vi "Execute.vi"(8 "error in":errorcluster, 9 "Consumer Queues in":T2, 10 "Trig Process Command in":refnum<class "TRIG Next Acq Request.lvclass">, 11 "Trig Process Data in":T1) -> (0 "error out":errorcluster, 1 "Consumer Queues out":T2, 2 "Stop?":bool, 3 "Trig Process Data out":T1)   [LabVIEW 2019, in "Trig Process.lvlib" / "TRIG Next Acq Request.lvclass"]
uses:
  TRIG Next Acq Request.lvclass
  TS Framework/Consumer Queues.ctl
  UI Process/Generic UI Command/Generic UI Process Command.lvclass
  DAC Process/Generic DAC Command/Generic DAC Process Command.lvclass
  Generic Trig Command/Generic Trig Process Command.lvclass
  Trig Process Data.ctl
  DAC Process/Start DAC/Start DAC.lvclass
  DAC Process/Start DAC/Start DAC.lvclass/Start DAC.ctl
  TS Framework/TS Framework.lvlib
  Trig Process.lvlib
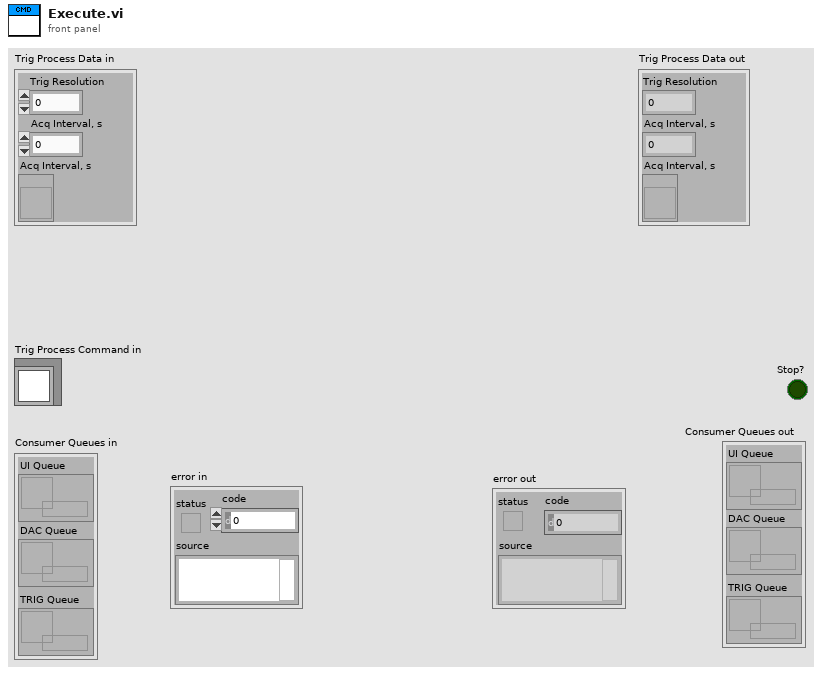
[diagram p1: front panel]
types:
  T1 = typedef "Trig Process.lvlib/Trig Process Data.ctl" = cluster{"Trig Resolution":u32, "Ctrl Interval":dbl, "Acq Interval":refnum<vi>}
  T2 = typedef "TS Framework.lvlib/Consumer Queues.ctl" = cluster{"UI Queue":refnum<queue>, "DAC Queue":refnum<queue>, "TRIG Queue":refnum<queue>}
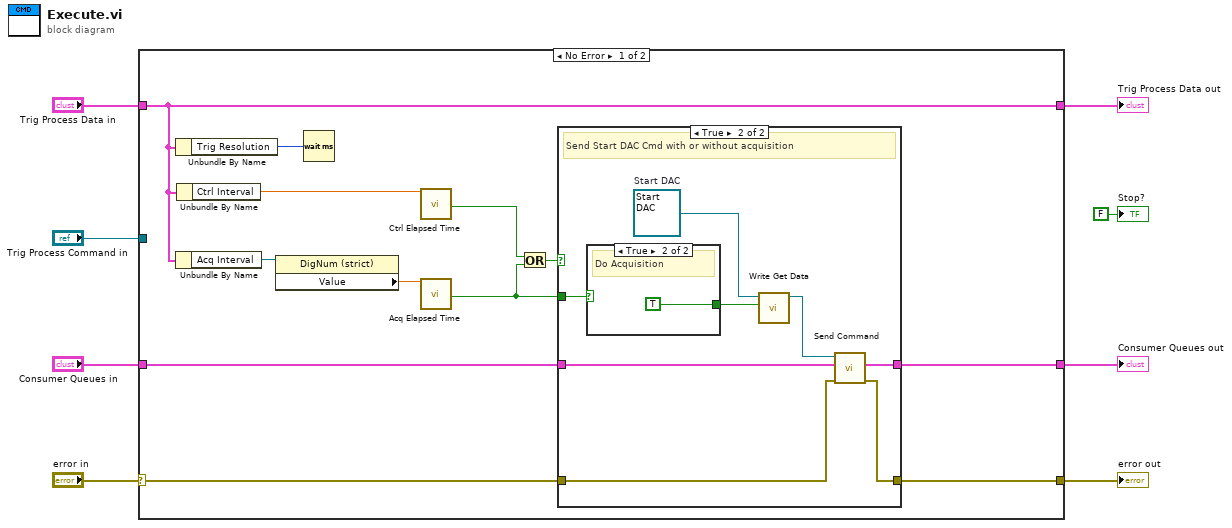
[diagram p0: block diagram]
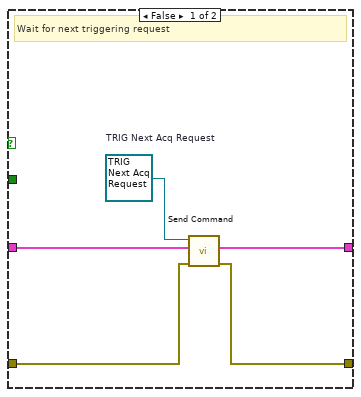
[diagram p2: hidden frame]
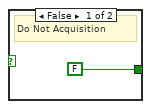
[diagram p3: hidden frame]
diagram:
  n1 = case shown="No Error" "error in" {
    selector: "error in" -> [w10 w38]
    tunnel: [w9 w38] -> w3
    tunnel: "Consumer Queues in" -> [w20 w37]
    tunnel: [w19 w37] -> w4
    tunnel: "Trig Process Data in" -> [w15 w36]
    tunnel: [w15 w36] -> w5
    tunnel: "Trig Process Command in" -> [_ _]
    frame No Error {
      n2 = Unbundle By Name(w15) -> ("Trig Resolution"=w17:u32)
      n3 = Unbundle By Name(w15) -> ("Acq Interval"=w14:refnum<vi>)
      n4 = Unbundle By Name(w15) -> ("Ctrl Interval"=w18:dbl)
      n5 = property class="DigNum (strict)"(reference=w14) -> ("Value"=w16:dbl)  [unwired: 1 in, 2 out]
      n6 = Wait (ms)(milliseconds to wait=w17) -> ()  [unwired: 1 out]
      n7 = call "Ctrl Elapsed Time"("Time Target (s)"=w18) -> ("Time has Elapsed"=w12:bool)  [unwired: 11 in, 7 out]
      n8 = call "Acq Elapsed Time"("Time Target (s)"=w16) -> ("Time has Elapsed"=w11:bool)  [unwired: 11 in, 7 out]
      n9 = Or(x=w12, y=w11) -> (x .or. y?=w13:bool)
      n10 = case shown="True" w13 {
        tunnel: w20 -> [w24 w33]
        tunnel: [w22 w32] -> w19
        tunnel: w11 -> [_ w28]
        tunnel: w10 -> [w23 w27]
        tunnel: [w21 w26] -> w9
        frame False {
          w25 = refnum<class "TRIG Next Acq Request.lvclass"> refnum  # TRIG Next Acq Request
          # "Wait for next triggering request"
          n11 = call-dynamic "Send Command.vi"("error in (no error)"=w23, "Consumer Queues in"=w24, "Trig Process Command"=w25) -> ("error out"=w21:errorcluster, "Consumer Queues out"=w22:T2)  [unwired: 7 in]
        }
        frame True {
          w31 = refnum<class "Start DAC.lvclass"> refnum  # Start DAC
          # "Send Start DAC Cmd with or without acquisition"
          n12 = case shown="True" w28 {
            tunnel: [FALSE TRUE] -> w29
            frame False {
              # "Do Not Acquisition"
            }
            frame True {
              # "Do Acquisition"
            }
          }
          n13 = call "Write Get Data.vi"("Get Data"=w29, "Start DAC in"=w31) -> ("Start DAC out"=w30:refnum<class "Start DAC.lvclass">)  [unwired: 8 in, 1 out]
          n14 = call-dynamic "Send Command.vi"("error in (no error)"=w27, "Consumer Queues in"=w33, "DAC Process Command"=w30) -> ("error out"=w26:errorcluster, "Consumer Queues out"=w32:T2)  [unwired: 7 in]
        }
      }
    }
    frame Error {
    }
  }
  "error out" <- w3
  "Consumer Queues out" <- w4
  "Trig Process Data out" <- w5
  "Stop?" <- FALSE ("Stop?")
